vi "Voltage input PID Autotuning Online.vi"() -> ()   [LabVIEW 2019]
uses:
  <vilib>/addons/control/pid/autopid.llb/PID Online Autotuning (Relay Feedback).vi
  <vilib>/addons/control/pid/pid.llb/PID Advanced (DBL).vi
  <vilib>/addons/control/pid/NI_PID_autopid.lvlib
  <vilib>/addons/control/pid/NI_PID_pid.lvlib
panel:
  out "Valve input voltage":dbl(graph)
  in  "Tab Control":enum32{"Instructions", "Plant Parameters"}(tab)
  in  "Instructions":string="Overview: This example demonstrates how to use the  PID Online Autotuning VI with the PID using the Relay Autotuning Technique.\nInstructions:\n1. Run the VI and wait until the process variable (PV) reaches near setpoint (SP).\n2.  On the PID Autotuning Design section, select the type of algorithm, type of controller and excitation amplitude for the 'open loop step response'. Then, click Autotune to start the process.\n3.  When the tuned PID gains do not change anymore or the tuning completed? flashes, the identification is done and you can accept new gains by pressing Accept gain and that will transfer the new gain to PID Gains.\n4. Click Autotune again to go back to the automatic control. You can try different options and repeat this process.\n5. Click Stop to stop the VI.\n"
  out "Plant Variable Gain":dbl=5.68817109595442
  out "Plant Variable Lag":dbl=1.4596237458843302
  in  "Load":dbl(slide) scale=0.0..10.0
  in  "Stop":bool
  out "SP and PV":cluster{"initial PV":dbl, "SP1:":dbl}(graph)={"initial PV"=50.98160323470328, "SP1:"=50.98039215686275}
  in  "Sampling Time dt (s)":dbl=0.05 min=0.001 step=0.01 format="%#.3p"
  in  "PID Gains":T1={"proportional gain (Kc)"=0.05, "integral time (Ti, min)"=0.0, "derivative time (Td, min)"=0.0} {"derivative time (Td, min)" format="%#.6g"; "integral time (Ti, min)" format="%#.6g"; "proportional gain (Kc)" format="%#.6g"}
  in  "SP:":dbl(slide)=28.758169934640524 min=0.0 max=0.0 scale=0.0..10.0
  out "PV:":dbl(slide)=28.4408554797721 scale=0.0..10.0
  in  "MV:":dbl(slide)=0.015865722743421174 scale=-100.0..100.0
  in  "Autotune":bool
  in  "Accept gain":bool
  out "MV":dbl(graph)=20.39115328927357
  out "tuned PID gains":T1={"proportional gain (Kc)"=1.9838195929127882, "integral time (Ti, min)"=0.01995856284686879, "derivative time (Td, min)"=0.0} {"derivative time (Td, min)" format="%#.6g"; "integral time (Ti, min)" format="%#.6g"; "proportional gain (Kc)" format="%#.6g"}
  in  "autotuning parameters":T2={"Type of Controller"=0, "relay cycles"=3, "relay amplitude"=1.0, "control specifications"=2, "PV noise level"=0.1} {"PV noise level" format="%.2f"; "control specifications" items=["fast", "normal", "slow"]; "relay amplitude" format="%.2f"; "Type of Controller" items=["P", "PI", "PID"]}
  in  "Reinitialize":bool
  in  "Automatic":bool=TRUE
  in  "alpha":dbl(slide)=0.49999999999999994 scale=0.0..1.0
  out "tuning completed?":bool
  in  "gamma":dbl(slide)=0.5102040816326531 scale=0.0..1.0
  # "Plant Simulated Parameters"
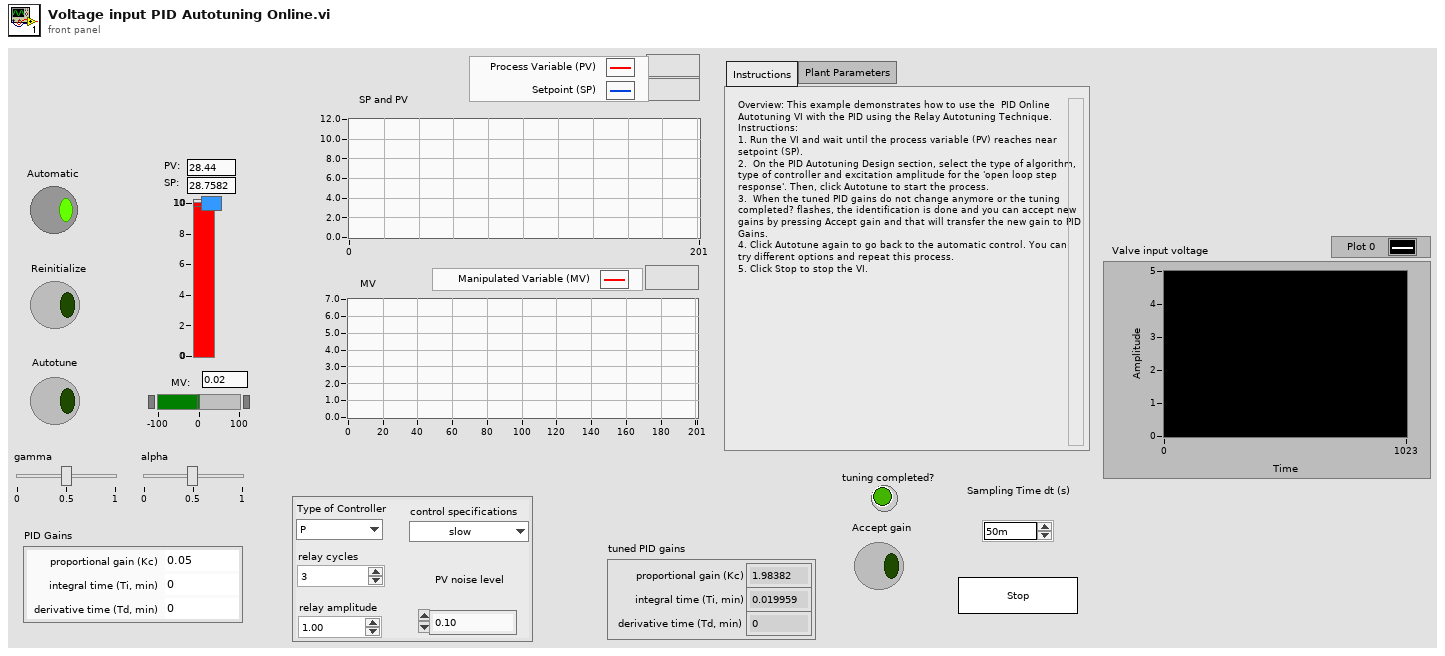
[diagram p1: front panel]
types:
  T1 = cluster{"proportional gain (Kc)":dbl, "integral time (Ti, min)":dbl, "derivative time (Td, min)":dbl}
  T2 = cluster{"Type of Controller":u16, "relay cycles":i32, "relay amplitude":dbl, "control specifications":u16, "PV noise level":dbl}
  T3 = cluster{"static gain":dbl, "lag (s)":dbl, "deadtime (s)":dbl, "load":dbl, "deadband":dbl, "sensor noise":dbl, "initial PV":dbl, "plant noise":dbl}
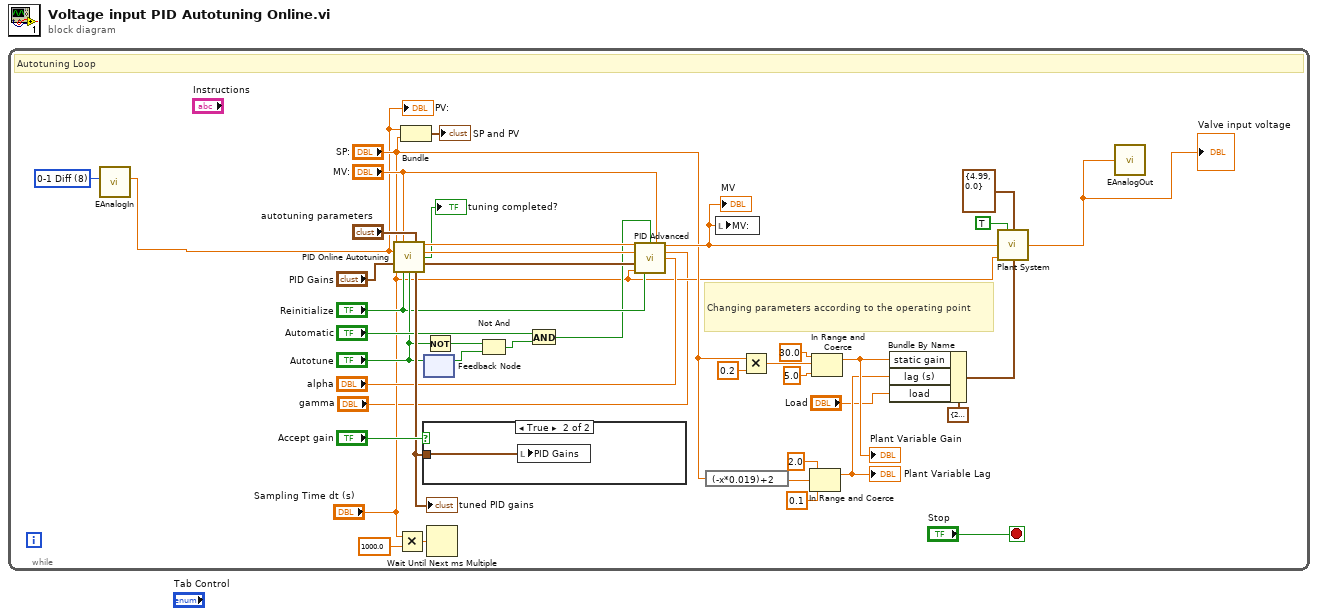
[diagram p0: block diagram]
diagram:
  n1 = while {
    stop <- "Stop" stop-if-true
    w2 = u16 8 items=["0 SE (+/-10V)", "1 SE (+/-10V)", "2 SE (+/-10V)", "3 SE (+/-10V)", "4 SE (+/-10V)", "5 SE (+/-10V)", "6 SE (+/-10V)", "7 SE (+/-10V)", "0-1 Diff", "2-3 Diff", "4-5 Diff", "6-7 Diff"] ("Channel")
    # "Changing parameters according to the operating point"
    # "Autotuning Loop"
    n2 = call <vilib>:"EAnalogIn.vi"("Channel"=w2) -> ("Voltage"=w1:dbl)  [unwired: 6 in, 4 out]
    "PV:" <- w1
    n3 = call-poly <vilib>:"PID Online Autotuning.VI"("setpoint"="SP:", "manipulated variable"="MV:", "autotuning parameters"="autotuning parameters", "process variable"=w1, "PID gains in"="PID Gains", "dt (s)"="Sampling Time dt (s)", "reinitialize? (F)"="Reinitialize", "autotune? (F)"="Autotune") -> ("setpoint out"=w32:dbl, "process variable out"=w31:dbl, "tuning completed?"=→"tuning completed?":bool, "PID gains out"=w27:T1, "tuned PID gains"=w26:T1)  [unwired: 3 in]
    "tuned PID gains" <- w26
    n4 = Multiply(x="Sampling Time dt (s)", y=1000.0) -> (x*y=w6:dbl)
    n5 = Bundle("Voltage"=w1, "SP:"="SP:") -> (→"SP and PV":cluster{"Voltage":dbl, "SP:":dbl})  [unwired: 1 in]
    n6 = case shown="True" "Accept gain" {
      tunnel: w26 -> [_ w43]
      frame False {
      }
      frame True {
        n7 = local write "PID Gains"(w43) -> ()
      }
    }
    n8 = feedback #1() -> (w22:bool)  [unwired: 1 in]
    n9 = feedback-in #1("Autotune") -> ()
    n10 = Not(x="Autotune") -> (.not. x?=w19:bool)
    n11 = Wait Until Next ms Multiple(millisecond multiple=w6) -> ()  [unwired: 1 out]
    n12 = Not And(1:w22, 2:w19) -> (0:w20:bool)
    n13 = And(x="Automatic", y=w20) -> (x .and. y?=w9:bool)
    n14 = call-poly <vilib>:"PID Advanced.vi"("setpoint"=w32, "auto? (T)"=w9, "manual control"="MV:", "process variable"=w31, "gamma"="gamma", "alpha"="alpha", "PID gains"=w27, "dt (s)"="Sampling Time dt (s)", "reinitialize? (F)"="Reinitialize") -> ("output"=w25:dbl)  [unwired: 5 in, 1 out]
    "MV" <- w25
    n15 = expression code="(-x*0.019)+2"("SP:") -> (w33:dbl)
    n16 = local write "MV:"(w25) -> ()
    n17 = Multiply(x="SP:", y=0.2) -> (x*y=w37:dbl)
    n18 = In Range and Coerce(upper limit=2.0, x=w33, lower limit=0.1) -> (coerced(x)=w14:dbl)  [unwired: 1 out]
    "Plant Variable Lag" <- w14
    n19 = In Range and Coerce(upper limit=30.0, x=w37, lower limit=5.0) -> (coerced(x)=w15:dbl)  [unwired: 1 out]
    "Plant Variable Gain" <- w15
    n20 = Bundle By Name(cluster=T3 {"static gain"=2.5, "lag (s)"=2.5, "deadtime (s)"=0.5, "load"=0.0, "deadband"=0.0, "sensor noise"=0.0, "initial PV"=30.0, "plant noise"=0.0} ("process parameters"), "static gain"=w15, "lag (s)"=w14, "load"="Load") -> (w5:T3)
    n21 = call "Plant System.vi"("Integrator ?"=TRUE, "output saturation range"=cluster{"output high":dbl, "output low":dbl} {"output high"=4.99, "output low"=0.0}, "Plant Input"=w25, "dt (s)"="Sampling Time dt (s)", "process parameters"=w5) -> ("Plant Output"=w3:dbl)  [unwired: 10 in]
    "Valve input voltage" <- w3
    n22 = call <vilib>:"EAnalogOut.vi"("Analog Output 0 [volts]"=w3) -> ()  [unwired: 13 in, 2 out]
  }
